vi "Test.vi"(10 "headless":bool, 11 "reportPath":path) -> (0 "error out":errorcluster, 3 "testsPassed":bool)   [LabVIEW 2026, in "Tests.lvlib"]
doc: "Caraya test-suite runner for Lumberjack. Runs the full test hierarchy headlessly and writes a report to reportPath, returning the aggregate pass/fail on error out (and testsPassed). Wraps Define Test Suite and Destroy Test Suite around the test cases; individual test VIs register their assertions within the suite scope. The single entry point for a regression run (Test-Strategy 6)."
uses:
  Tests.lvlib
  <vilib>/addons/_JKI Toolkits/Caraya/classes/Test Suite/Define Test Suite (SimpleText Report).vi
  <vilib>/addons/_JKI Toolkits/Caraya/classes/Test Suite/Test Suite.lvclass
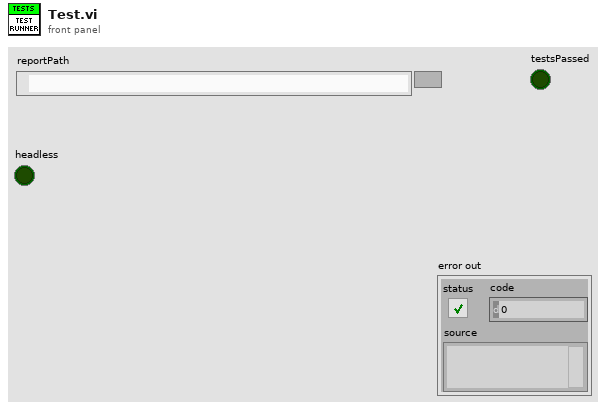
[diagram p1: front panel]
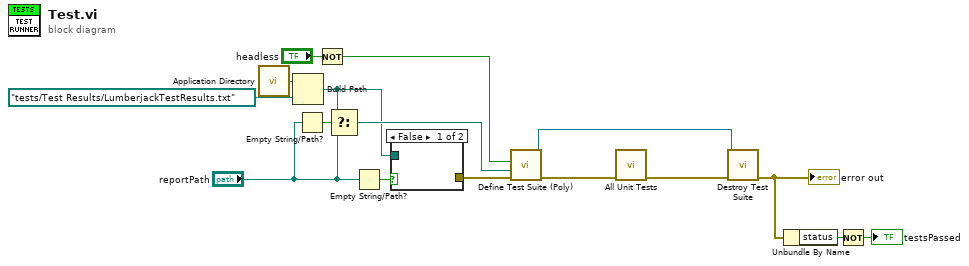
[diagram p0: block diagram]
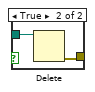
[diagram p2: hidden frame]
diagram:
  n1 = call <vilib>:"Application Directory.vi"() -> ("Application Directory"=w12:path)
  n2 = Build Path(base path=w12, name or relative path=path "tests/Test Results/LumberjackTestResults.txt") -> (appended path=w1:path)
  n3 = Empty String/Path?(string/path="reportPath") -> (empty?=w10:bool)
  n4 = Not(x="headless") -> (.not. x?=w6:bool)
  n5 = Select(t=w1, s=w10, f="reportPath") -> (s? t:f=w11:path)
  n6 = Empty String/Path?(string/path="reportPath") -> (empty?=w3:bool)
  n7 = case shown="False" w3 {
    tunnel: w1 -> [_ w18]
    tunnel: [_ w17] -> w4
    frame False {
    }
    frame True {
      n8 = Delete(path (use dialog)=w18) -> (error out=w17:errorcluster)  [unwired: 4 in, 2 out]
    }
  }
  n9 = call-poly <vilib>:"Define Test Suite (Poly).vi"("error in (no error)"=w4, "Report Path"=w11, "Interactive"=w6) -> ("error out"=w9:errorcluster, "Test Suite"=w16:refnum<class "Test Suite.lvclass">)  [unwired: 6 in, 1 out]
  n10 = call "All Unit Tests.vi"("error in (no error)"=w9) -> ("error out"=w8:errorcluster)  [unwired: 10 in]
  n11 = call-dynamic "Destroy Test Suite.vi"("error in (no error)"=w8, "Test Suite in"=w16) -> ("error out"=w15:errorcluster)  [unwired: 8 in, 1 out]
  "error out" <- w15
  n12 = Unbundle By Name(w15) -> ("status"=w14:bool)
  n13 = Not(x=w14) -> (.not. x?=→"testsPassed":bool)
